vi "WAFL Demo.vi"(6 "Variant in":variant, 7 "Shift Pressed?":bool, 8 "error in (no error)":errorcluster, 10 "QD Combo Box Ref":refnum<vi>, 11 "QD Launch VI Ref":refnum<vi>) -> (0 "error out":errorcluster, 4 "Variant out":variant)   [LabVIEW 2019]
doc: "Vertical Compress or distribute\n\nDefault Shortcut - [j]"
panel:
  in  "Undo Name":string="WAFL Demo"
  # "Do not change the connector pane of this VI.\n\nSee the block diagram for directions on how to use this template."
  # "Specify the name of the Undo transaction"
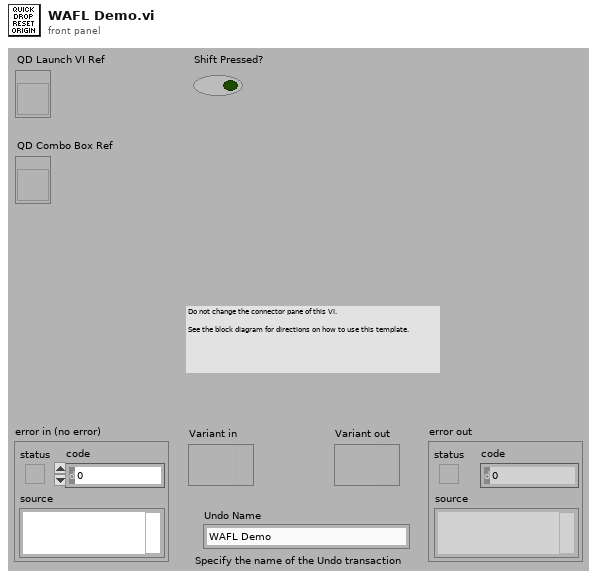
[diagram p1: front panel]
types:
  T1 = enum32{"Top Edges", "Vertical Centers", "Bottom Edges", "Vertical Gap", "Vertical Compress", "Left Edges", "Horizontal Centers", "Right Edges", "Horizontal Gap", "Horizontal Compress"}
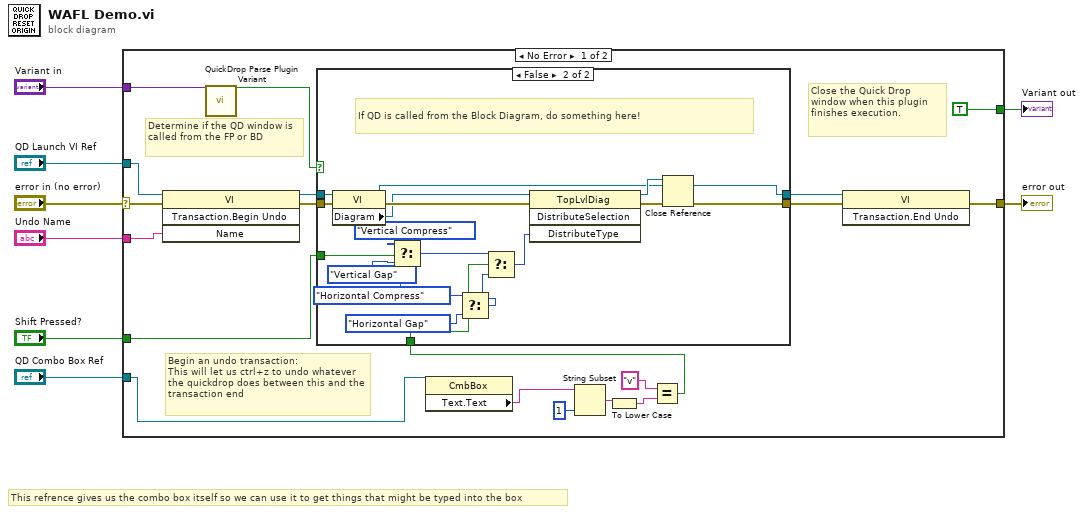
[diagram p0: block diagram]
diagram:
  # "This refrence gives us the combo box itself so we can use it to get things that might be typed into the box"
  n1 = case shown="No Error" "error in (no error)" {
    selector: "error in (no error)" -> [w26 w47]
    tunnel: [w20 w47] -> w7
    tunnel: "QD Launch VI Ref" -> [w25 _]
    tunnel: "Shift Pressed?" -> [w16 _]
    tunnel: "QD Combo Box Ref" -> [w15 _]
    tunnel: "Variant in" -> [w27 _]
    tunnel: "Undo Name" -> [w24 _]
    tunnel: [TRUE _] -> w1
    frame No Error {
      # "Begin an undo transaction:\nThis will let us ctrl+z to undo whatever the quickdrop does between this and the transaction end"
      # "Close the Quick Drop window when this plugin finishes execution."
      # "Determine if the QD window is called from the FP or BD"
      n2 = invoke class="VI" method="Transaction.Begin Undo"(reference=w25, error in=w26, "Name"=w24) -> (reference out=w19:refnum<vi>, error out=w21:errorcluster)  [unwired: 1 in, 2 out]
      n3 = call <vilib>:"QuickDrop Parse Plugin Variant.vi"("QDKS Variant in"=w27) -> ("QD Launch VI Panel?"=w22:bool)  [unwired: 12 in, 2 out]
      n4 = property class="CmbBox"(reference=w15) -> ("Text.Text"=w14:string)  [unwired: 1 in, 2 out]
      n5 = String Subset(string=w14, length (rest)=1 ("length (rest)")) -> (substring=w12:string)  [unwired: 1 in]
      n6 = To Lower Case(string=w12) -> (all lower case string=w11:string)
      n7 = Equal?(x="v", y=w11) -> (x = y?=w9:bool)
      n8 = case shown="False" w22 {
        tunnel: w21 -> [w28 w45]
        tunnel: w19 -> [w29 w46]
        tunnel: [w28 w42] -> w18
        tunnel: [w29 w31] -> w17
        tunnel: w16 -> [_ w32]
        tunnel: w9 -> [_ w38]
        frame True {
          # "If QD is called from the Front Panel, do something here!"
        }
        frame False {
          # "If QD is called from the Block Diagram, do something here!"
          n9 = property class="VI"(reference=w46, error in=w45) -> (reference out=w31:refnum<vi>, error out=w44:errorcluster, "Diagram"=w30:refnum<vi>)
          n10 = Select(t=T1."Vertical Compress" ("DistributeType"), s=w32, f=T1."Vertical Gap" ("DistributeType")) -> (s? t:f=w40:T1)
          n11 = Select(t=T1."Horizontal Compress" ("DistributeType"), s=w32, f=T1."Horizontal Gap" ("DistributeType")) -> (s? t:f=w33:T1)
          n12 = Select(t=w40, s=w38, f=w33) -> (s? t:f=w39:T1)
          n13 = invoke class="TopLvlDiag" method="DistributeSelection"(reference=w30, error in=w44, "DistributeType"=w39) -> (reference out=w41:refnum<vi>, error out=w43:errorcluster)  [unwired: 1 in, 2 out]
          n14 = Close Reference(reference=w41, error in (no error)=w43) -> (error out=w42:errorcluster)
        }
      }
      n15 = invoke class="VI" method="Transaction.End Undo"(reference=w17, error in=w18) -> (error out=w20:errorcluster)  [unwired: 1 in, 2 out]
    }
    frame Error {
    }
  }
  "error out" <- w7
  "Variant out" <- w1
